vi "HW5p1_Task2_nguyejk.vi"() -> ()   [LabVIEW 2016]
panel:
  out "Diastolic":string
  out "Most severe":string
  out "Systolic":string
  in  "Diastolic":dbl
  in  "Systolic":dbl
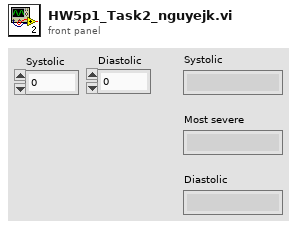
[diagram p1: front panel]
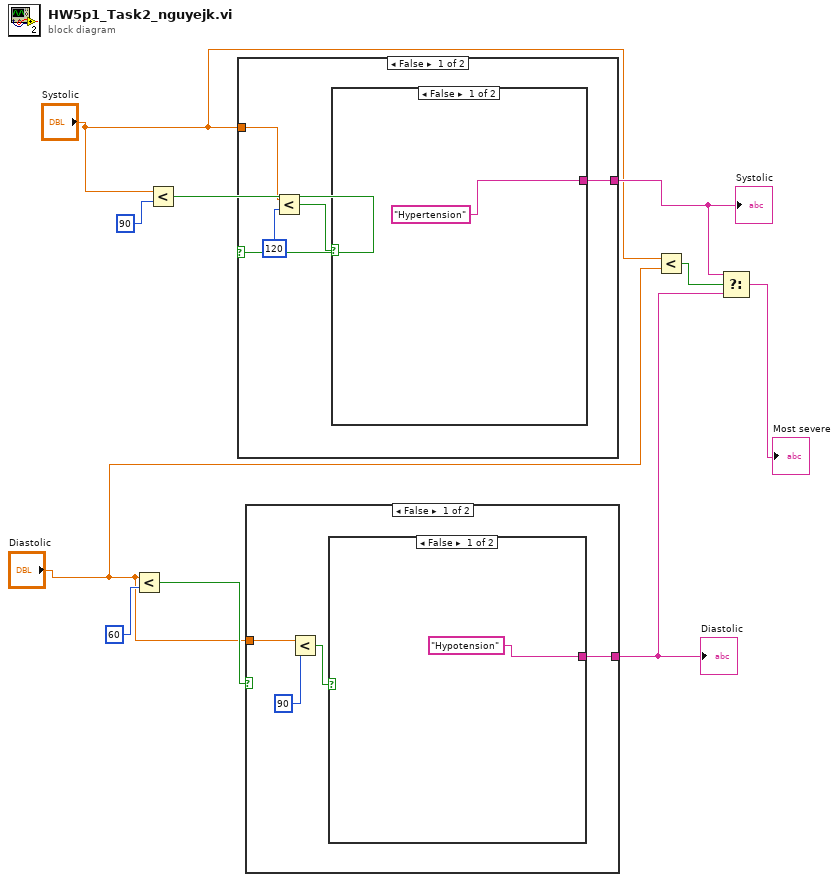
[diagram p0: block diagram]
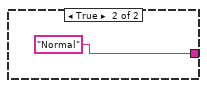
[diagram p2: hidden frame]
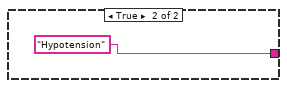
[diagram p3: hidden frame]
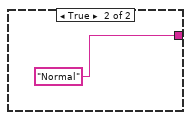
[diagram p4: hidden frame]
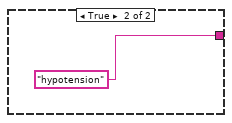
[diagram p5: hidden frame]
diagram:
  n1 = Less?(x="Diastolic", y=60) -> (x < y?=w7:bool)
  n2 = Less?(x="Systolic", y=90) -> (x < y?=w9:bool)
  n3 = case shown="False" w9 {
    tunnel: [w12 "hypotension"] -> w6
    tunnel: "Systolic" -> [w11 _]
    frame False {
      n4 = Less?(x=w11, y=120) -> (x < y?=w13:bool)
      n5 = case shown="False" w13 {
        tunnel: ["Hypertension" "Normal"] -> w12
        frame False {
        }
        frame True {
        }
      }
    }
    frame True {
    }
  }
  "Systolic" <- w6
  n6 = case shown="False" w7 {
    tunnel: [w18 "Hypotension"] -> w5
    tunnel: "Diastolic" -> [w20 _]
    frame False {
      n7 = Less?(x=w20, y=90) -> (x < y?=w19:bool)
      n8 = case shown="False" w19 {
        tunnel: ["Hypotension" "Normal"] -> w18
        frame False {
        }
        frame True {
        }
      }
    }
    frame True {
    }
  }
  "Diastolic" <- w5
  n9 = Less?(x="Systolic", y="Diastolic") -> (x < y?=w1:bool)
  n10 = Select(t=w6, s=w1, f=w5) -> (s? t:f=→"Most severe":string)
